vi "Get Owner Enqueuer from Sync DVR.vi"(8 "error in (no error)":errorcluster, 11 "Data Value Reference in":refnum<data-value>) -> (0 "error out":errorcluster, 2 "Owner Enqueuer":refnum<class "Message Enqueuer.lvclass">, 3 "Data Value Reference out":refnum<data-value>)   [LabVIEW 2020, in "Instrument Handler.lvlib" / "Instrument Handler.lvclass"]
doc: "Extract the Owner Enqueuer from the Sync DVR."
uses:
  Instrument Handler.lvclass
  PPL/HDH.Actor Framework.Core.Actor.lvlibp/1abvi3w/vi.lib/ActorFramework/Message Enqueuer/Message Enqueuer.lvclass
  Controls/Ctl_InstrumentSynchronicationCluster.ctl
  PPL/HDH.Actor Framework.Core.Instrument Driver.lvlibp/Instrument Driver/Controls/Ctl_ConnectionType.ctl
  PPL/HDH.Data.Generic.lvlibp/Synchronization/Notifier/Notifier.lvclass
  PPL/HDH.Actor Framework.Core.Sequencer.lvlibp/Sequencer Core/Sequencer Core.lvclass
  PPL/HDH.Actor Framework.Core.Instrument Driver.lvlibp/Instrument Driver/Instrument Driver.lvclass
  Instrument Handler.lvlib
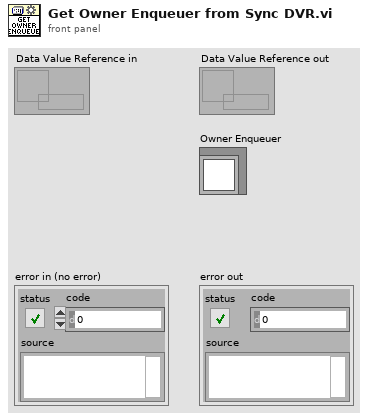
[diagram p1: front panel]
types:
  T1 = typedef "Instrument Handler.lvlib/Ctl_InstrumentSynchronicationCluster.ctl" = cluster{"Launched?":bool, "Driver Path":path, "Alias":string, "Connection Type":T2, "Pre Initialization Data":variant, "Enqueue Sync":refnum<class "Notifier.lvclass">, "Enqueue Lock":T3, "Owner Enqueuer":refnum<class "Message Enqueuer.lvclass">, "Owner":refnum<class "Sequencer Core.lvclass">, "Instrument ID":u32}
  T2 = typedef "HDH.Actor Framework.Core.Instrument Driver.lvlibp/Instrument Driver.lvclass/Ctl_ConnectionType.ctl" = enum16{"BuiltIn/System", "PXI/PCI", "USB", "GPIB", "VXI", "Serial", "TCP/IP", "cRIO", "SCXI", "cDAQ", "SwitchBlock", "SCC", "FireWire", "Accessory", "CAN", "SwitchBlock Device"}
  T3 = typedef "Semaphore RefNum" = refnum<k1>
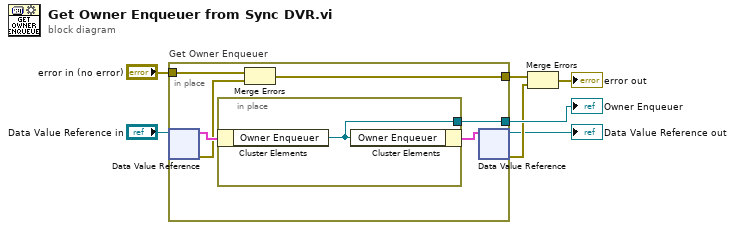
[diagram p0: block diagram]
diagram:
  n1 = in-place "Get Owner Enqueuer" {
    in-place-border: "error in (no error)" -> [w11]
    in-place-border: [w9] -> w4
    in-place-border: [w8] -> w7
    n2 = in-place-dvr #1("Data Value Reference in") -> (w13:T1, w10:errorcluster)
    n3 = in-place {
      in-place-border: [w14] -> w8
      n4 = in-place-cluster #2(w13) -> ("Owner Enqueuer"=w14:refnum<class "Message Enqueuer.lvclass">)
      n5 = in-place-cluster #2("Owner Enqueuer"=w14) -> (w12:T1)
    }
    n6 = Merge Errors(w11, w10) -> (w9:errorcluster)
    n7 = in-place-dvr #1(w12) -> (→"Data Value Reference out":refnum<data-value>, w5:errorcluster)
  }
  "Owner Enqueuer" <- w7
  n8 = Merge Errors(w4, w5) -> (→"error out":errorcluster)
